vi "toGroupView.vi"(11 "tagbus":cluster{"read":T4, "write":T4}) -> (3 "GroupTags":T1[](array[typedef]))   [LabVIEW 2013]
uses:
  <vilib>/NI/Tag Bus/dictionary/full data dictionary.ctl
  GroupTags.ctl
  TypeTags.ctl
  TagPermission.ctl
  <vilib>/NI/Tag Bus/dictionary/data dictionary.lvclass
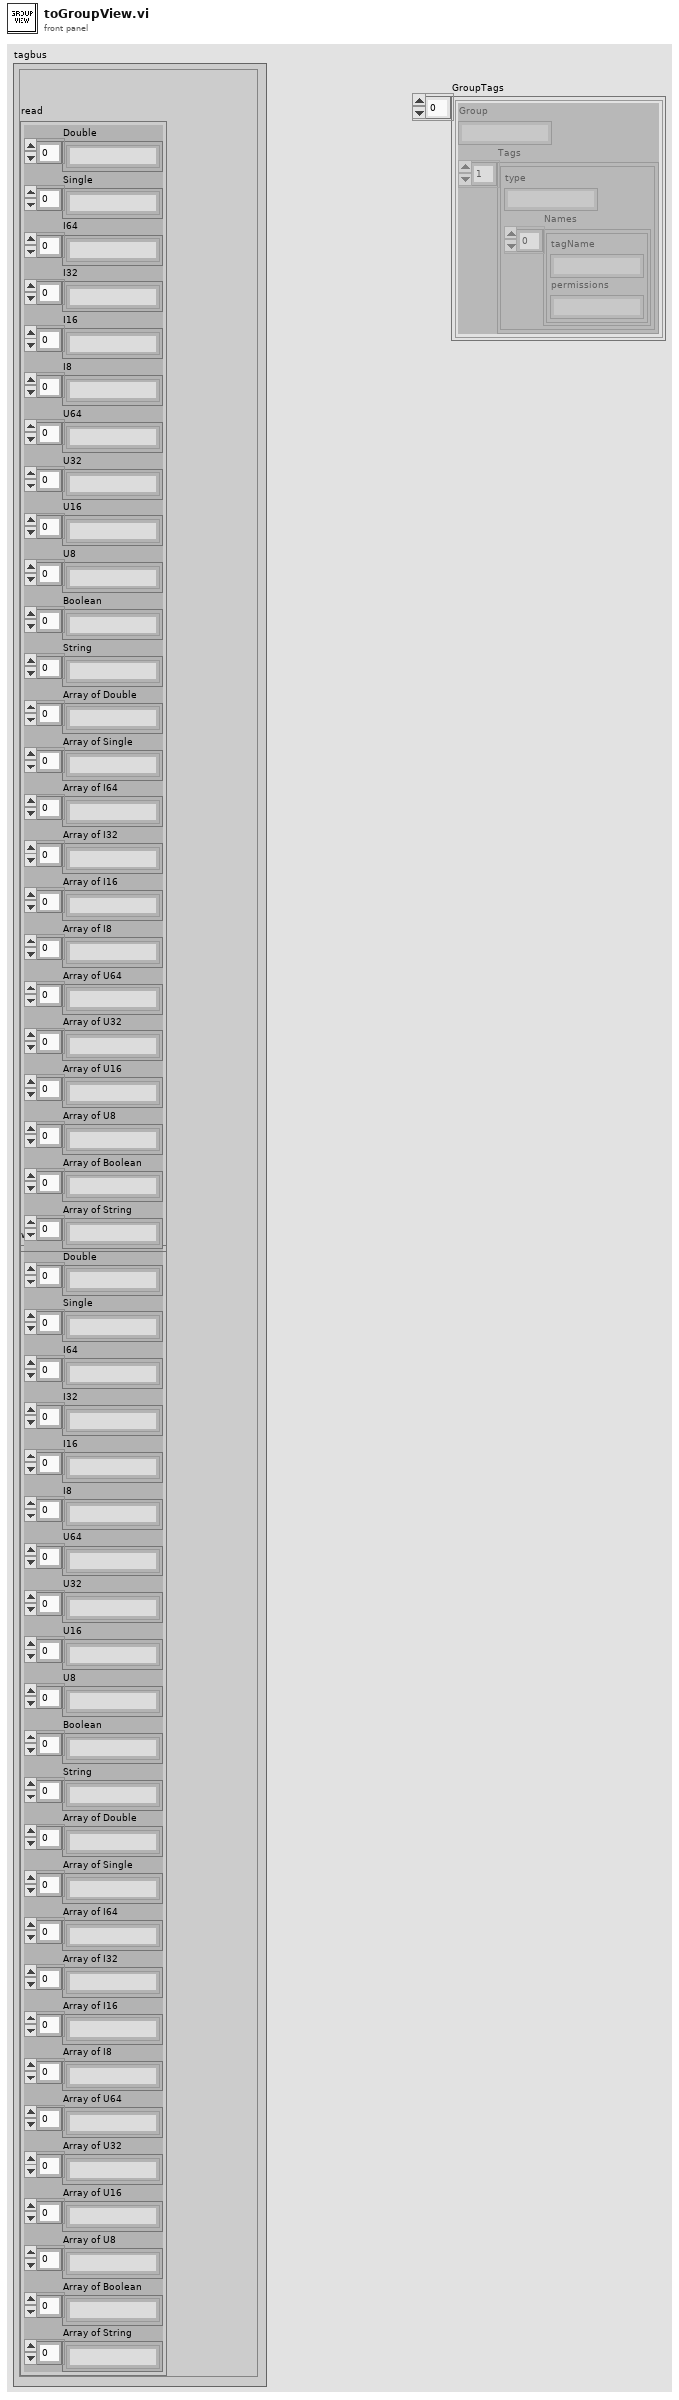
[diagram p1: front panel]
types:
  T1 = typedef "GroupTags.ctl" = cluster{"Group":string, "Tags":T2[]}
  T2 = typedef "TypeTags.ctl" = cluster{"type":string, "Names":T3[]}
  T3 = typedef "TagPermission.ctl" = cluster{"tagName":string, "permissions":string}
  T4 = typedef "tag bus.lvlib/data dictionary.lvclass/full data dictionary.ctl" = cluster{"Double":string[], "Single":string[], "I64":string[], "I32":string[], "I16":string[], "I8":string[], "U64":string[], "U32":string[], "U16":string[], "U8":string[], "Boolean":string[], "String":string[], "Array of Double":string[], "Array of Single":string[], "Array of I64":string[], "Array of I32":string[], "Array of I16":string[], "Array of I8":string[], "Array of U64":string[], "Array of U32":string[], "Array of U16":string[], "Array of U8":string[], "Array of Boolean":string[], "Array of String":string[]}
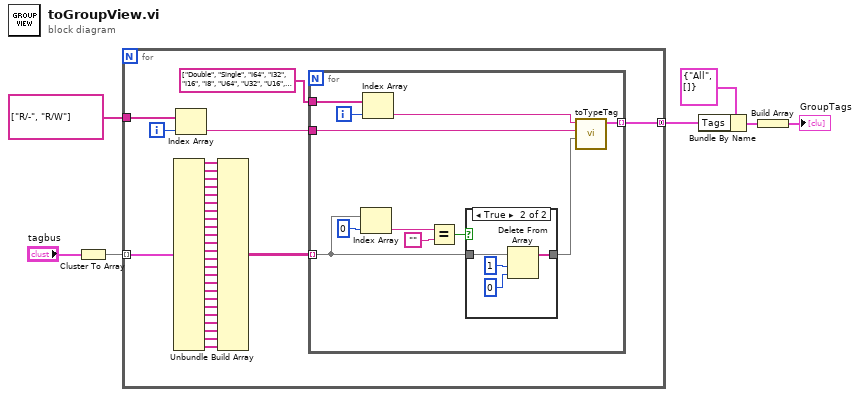
[diagram p0: block diagram]
diagram:
  n1 = Cluster To Array(cluster="tagbus") -> (array=w7:T4[])
  n2 = for {
    tunnel: w7 -> [w38] mode=indexing
    tunnel: string[] ["R/-", "R/W"] -> [w12]
    tunnel: [w9] -> w3 mode=concatenating
    i -> [w8]
    n3 = Unbundle(w38) -> ("Double"=w37:string[], "Single"=w36:string[], "I64"=w35:string[], "I32"=w34:string[], "I16"=w33:string[], "I8"=w32:string[], "U64"=w31:string[], "U32"=w30:string[], "U16"=w29:string[], "U8"=w28:string[], "Boolean"=w27:string[], "String"=w26:string[], "Array of Double"=w25:string[], "Array of Single"=w24:string[], "Array of I64"=w23:string[], "Array of I32"=w22:string[], "Array of I16"=w21:string[], "Array of I8"=w20:string[], "Array of U64"=w19:string[], "Array of U32"=w18:string[], "Array of U16"=w17:string[], "Array of U8"=w16:string[], "Array of Boolean"=w15:string[], "Array of String"=w14:string[])
    n4 = Index Array(array=w12, index=w8) -> (element=w11:string)
    n5 = Build Array(w37, w36, w35, w34, w33, w32, w31, w30, w29, w28, w27, w26, w25, w24, w23, w22, w21, w20, w19, w18, w17, w16, w15, w14) -> (w13:string[][])
    n6 = for {
      tunnel: w13 -> [w40] mode=indexing
      tunnel: w11 -> [w49]
      tunnel: string[] ["Double", "Single", "I64", "I32", "I16", "I8", "U64", "U32", "U16", "U8", "Boolean", "String"] -> [w48]
      tunnel: [w46] -> w9 mode=indexing
      i -> [w45]
      n7 = Index Array(array=w40, index=0) -> (element=w43:string)
      n8 = Index Array(array=w48, index=w45) -> (element=w47:string)
      n9 = Equal?(x=w43, y="") -> (x = y?=w41:bool)
      n10 = case shown="True" w41 {
        tunnel: w40 -> [w50 w54]
        tunnel: [w50 w51] -> w39
        frame False {
        }
        frame True {
          n11 = Delete From Array(array=w54, length=1, index=0) -> (array with subset deleted=w51:string[])  [unwired: 1 out]
        }
      }
      n12 = call "toTypeTag.vi"("Tags"=w39, "permission"=w49, "type"=w47) -> ("typeTags"=w46:T2)  [unwired: 8 in]
    }
  }
  n13 = Bundle By Name(cluster=T1 {"Group"="All", "Tags"=[]} ("GroupTags"), "Tags"=w3) -> (w5:T1)
  n14 = Build Array(w5) -> (→"GroupTags":T1[])
